vi "ParseSlaveRWw.vi"(0 "Node RWw":u16[][](array[numeric])) -> (1 "当前档位":sgl, 2 "PLC采集值":T2, 3 "PLC档位序号":T1, 4 "行号":i32)   [LabVIEW 2018]
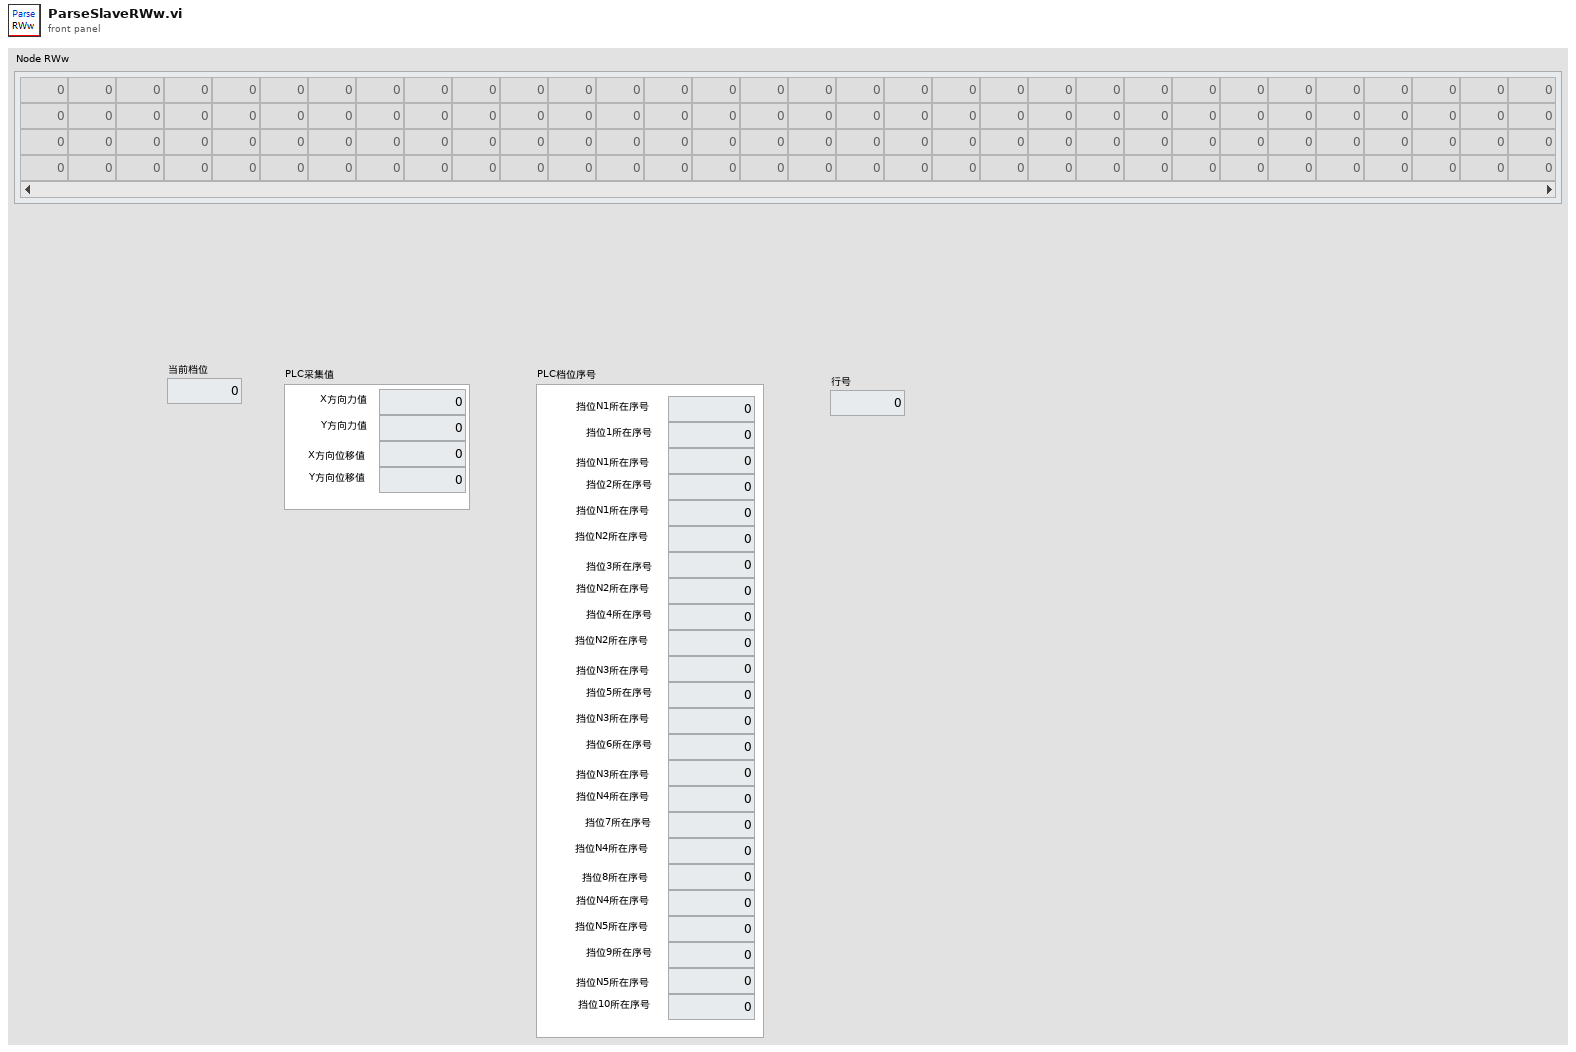
[diagram p1: front panel]
types:
  T1 = cluster{"挡位N1所在序号":sgl, "挡位1所在序号":sgl, "挡位N1所在序号":sgl, "挡位2所在序号":sgl, "挡位N1所在序号":sgl, " 挡位N2所在序号":sgl, "挡位3所在序号":sgl, "挡位N2所在序号":sgl, "挡位4所在序号":sgl, " 挡位N2所在序号":sgl, "挡位N3所在序号":sgl, "挡位5所在序号":sgl, "挡位N3所在序号":sgl, "挡位6所在序号":sgl, "挡位N3所在序号":sgl, "挡位N4所在序号":sgl, " 挡位7所在序号":sgl, " 挡位N4所在序号":sgl, "挡位8所在序号":sgl, "挡位N4所在序号":sgl, " 挡位N5所在序号":sgl, "挡位9所在序号":sgl, "挡位N5所在序号":sgl, " 挡位10所在序号":sgl}
  T2 = cluster{"X方向力值":sgl, "Y方向力值":sgl, "X方向位移值":sgl, "Y方向位移值":sgl}
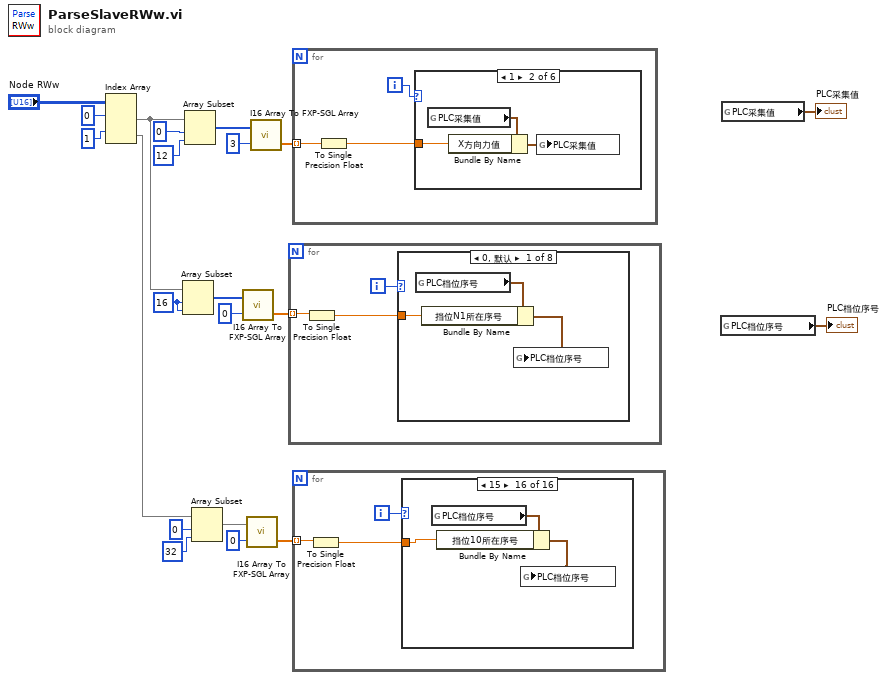
[diagram p0: block diagram]
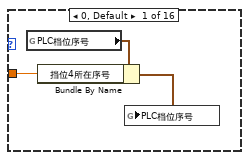
[diagram p2: hidden frame]
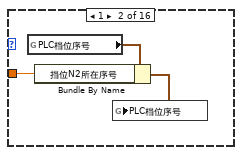
[diagram p3: hidden frame]
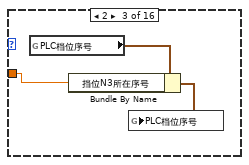
[diagram p4: hidden frame]
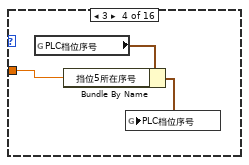
[diagram p5: hidden frame]
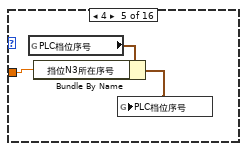
[diagram p6: hidden frame]
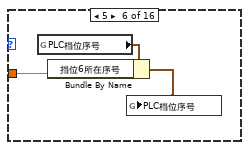
[diagram p7: hidden frame]
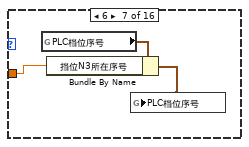
[diagram p8: hidden frame]
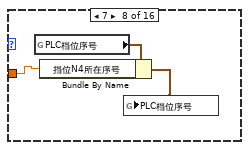
[diagram p9: hidden frame]
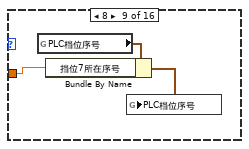
[diagram p10: hidden frame]
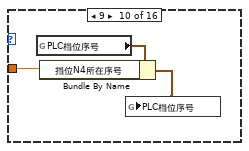
[diagram p11: hidden frame]
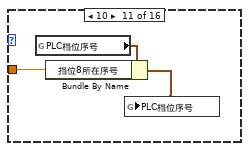
[diagram p12: hidden frame]
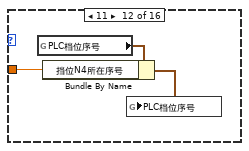
[diagram p13: hidden frame]
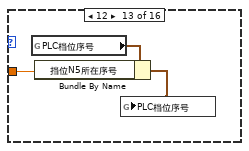
[diagram p14: hidden frame]
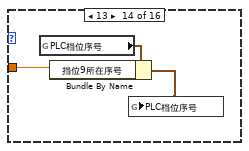
[diagram p15: hidden frame]
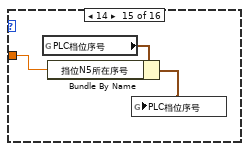
[diagram p16: hidden frame]
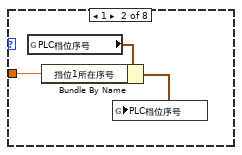
[diagram p17: hidden frame]
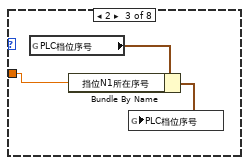
[diagram p18: hidden frame]
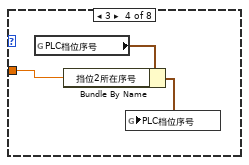
[diagram p19: hidden frame]
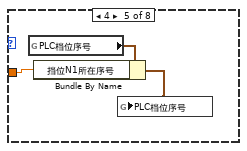
[diagram p20: hidden frame]
diagram:
  w11 = 16 ("索引")
  n1 = Index Array(array="Node RWw", index (row) #1=0 ("索引 (行)"), index (row) #2=1 ("索引 (行)")) -> (element #1=w12:u16[], element #2=w6:u16[])  [unwired: 2 in]
  n2 = Array Subset(array=w12, index=w11, length=w11) -> (w10:u16[])
  n3 = Array Subset(array=w12, index=0 ("索引"), length=12 ("长度")) -> (w15:u16[])
  n4 = Array Subset(array=w6, index=0 ("索引"), length=32 ("长度")) -> (w3:u16[])
  n5 = call "I16 Array To FXP-SGL Array.vi"("小数位数"=0, "I16 Array"=w10) -> ("SGL Array"=w8:sgl[])  [unwired: 1 out]
  n6 = call "I16 Array To FXP-SGL Array.vi"("小数位数"=0, "I16 Array"=w3) -> ("SGL Array"=w1:sgl[])  [unwired: 1 out]
  n7 = call "I16 Array To FXP-SGL Array.vi"("小数位数"=3, "I16 Array"=w15) -> ("SGL Array"=w18:sgl[])  [unwired: 1 out]
  n8 = for {
    tunnel: w8 -> [w24] mode=indexing
    i -> [w23]
    n9 = To Single Precision Float(number=w24) -> (single precision float=w22:sgl)
    n10 = case shown="0, 默认" w23 {
      tunnel: w22 -> [w26 w30 w32 w35 w39 w40 w43 w46]
      frame 0, Default {
        n11 = global read "全局 1.vi" "PLC档位序号"() -> (w27:T1)
        n12 = Bundle By Name(cluster=w27, "挡位N1所在序号"=w26) -> (w25:T1)
        n13 = global write "全局 1.vi" "PLC档位序号"(w25) -> ()
      }
      frame 1 {
        n14 = global read "全局 1.vi" "PLC档位序号"() -> (w29:T1)
        n15 = Bundle By Name(cluster=w29, "挡位1所在序号"=w30) -> (w28:T1)
        n16 = global write "全局 1.vi" "PLC档位序号"(w28) -> ()
      }
      frame 2 {
        n17 = global read "全局 1.vi" "PLC档位序号"() -> (w33:T1)
        n18 = Bundle By Name(cluster=w33, "挡位N1所在序号"=w32) -> (w31:T1)
        n19 = global write "全局 1.vi" "PLC档位序号"(w31) -> ()
      }
      frame 3 {
        n20 = global read "全局 1.vi" "PLC档位序号"() -> (w36:T1)
        n21 = Bundle By Name(cluster=w36, "挡位2所在序号"=w35) -> (w34:T1)
        n22 = global write "全局 1.vi" "PLC档位序号"(w34) -> ()
      }
      frame 4 {
        n23 = global read "全局 1.vi" "PLC档位序号"() -> (w38:T1)
        n24 = Bundle By Name(cluster=w38, "挡位N1所在序号"=w39) -> (w37:T1)
        n25 = global write "全局 1.vi" "PLC档位序号"(w37) -> ()
      }
      frame 5 {
        n26 = global read "全局 1.vi" "PLC档位序号"() -> (w42:T1)
        n27 = Bundle By Name(cluster=w42, "挡位N2所在序号"=w40) -> (w41:T1)
        n28 = global write "全局 1.vi" "PLC档位序号"(w41) -> ()
      }
      frame 6 {
        n29 = global read "全局 1.vi" "PLC档位序号"() -> (w45:T1)
        n30 = Bundle By Name(cluster=w45, "挡位3所在序号"=w43) -> (w44:T1)
        n31 = global write "全局 1.vi" "PLC档位序号"(w44) -> ()
      }
      frame 7 {
        n32 = global read "全局 1.vi" "PLC档位序号"() -> (w48:T1)
        n33 = Bundle By Name(cluster=w48, "挡位N2所在序号"=w46) -> (w47:T1)
        n34 = global write "全局 1.vi" "PLC档位序号"(w47) -> ()
      }
    }
  }
  n35 = for {
    tunnel: w18 -> [w51] mode=indexing
    i -> [w49]
    n36 = To Single Precision Float(number=w51) -> (single precision float=w50:sgl)
    n37 = case shown="1" w49 {
      tunnel: w50 -> [w54 w57 w60 w63 w66 w69]
      frame 0, Default {
        n38 = Multiply(x=w54, y=sgl 1000.0) -> (x*y=→"当前档位":sgl)
      }
      frame 1 {
        n39 = global read "全局 1.vi" "PLC采集值"() -> (w55:T2)
        n40 = Bundle By Name(cluster=w55, "X方向力值"=w57) -> (w56:T2)
        n41 = global write "全局 1.vi" "PLC采集值"(w56) -> ()
      }
      frame 2 {
        n42 = global read "全局 1.vi" "PLC采集值"() -> (w58:T2)
        n43 = Bundle By Name(cluster=w58, "Y方向力值"=w60) -> (w59:T2)
        n44 = global write "全局 1.vi" "PLC采集值"(w59) -> ()
      }
      frame 3 {
        n45 = global read "全局 1.vi" "PLC采集值"() -> (w61:T2)
        n46 = Bundle By Name(cluster=w61, "X方向位移值"=w63) -> (w62:T2)
        n47 = global write "全局 1.vi" "PLC采集值"(w62) -> ()
      }
      frame 4 {
        n48 = global read "全局 1.vi" "PLC采集值"() -> (w64:T2)
        n49 = Bundle By Name(cluster=w64, "Y方向位移值"=w66) -> (w65:T2)
        n50 = global write "全局 1.vi" "PLC采集值"(w65) -> ()
      }
      frame 5 {
        n51 = Multiply(x=w69, y=sgl 1000.0) -> (x*y=→"行号":sgl)
      }
    }
  }
  n52 = for {
    tunnel: w1 -> [w72] mode=indexing
    i -> [w71]
    n53 = To Single Precision Float(number=w72) -> (single precision float=w70:sgl)
    n54 = case shown="15" w71 {
      tunnel: w70 -> [w74 w78 w80 w83 w87 w88 w91 w94 w97 w100 w103 w106 w109 w112 w115 w118]
      frame 0, Default {
        n55 = global read "全局 1.vi" "PLC档位序号"() -> (w75:T1)
        n56 = Bundle By Name(cluster=w75, "挡位4所在序号"=w74) -> (w73:T1)
        n57 = global write "全局 1.vi" "PLC档位序号"(w73) -> ()
      }
      frame 1 {
        n58 = global read "全局 1.vi" "PLC档位序号"() -> (w77:T1)
        n59 = Bundle By Name(cluster=w77, "挡位N2所在序号"=w78) -> (w76:T1)
        n60 = global write "全局 1.vi" "PLC档位序号"(w76) -> ()
      }
      frame 2 {
        n61 = global read "全局 1.vi" "PLC档位序号"() -> (w81:T1)
        n62 = Bundle By Name(cluster=w81, "挡位N3所在序号"=w80) -> (w79:T1)
        n63 = global write "全局 1.vi" "PLC档位序号"(w79) -> ()
      }
      frame 3 {
        n64 = global read "全局 1.vi" "PLC档位序号"() -> (w84:T1)
        n65 = Bundle By Name(cluster=w84, "挡位5所在序号"=w83) -> (w82:T1)
        n66 = global write "全局 1.vi" "PLC档位序号"(w82) -> ()
      }
      frame 4 {
        n67 = global read "全局 1.vi" "PLC档位序号"() -> (w86:T1)
        n68 = Bundle By Name(cluster=w86, "挡位N3所在序号"=w87) -> (w85:T1)
        n69 = global write "全局 1.vi" "PLC档位序号"(w85) -> ()
      }
      frame 5 {
        n70 = global read "全局 1.vi" "PLC档位序号"() -> (w90:T1)
        n71 = Bundle By Name(cluster=w90, "挡位6所在序号"=w88) -> (w89:T1)
        n72 = global write "全局 1.vi" "PLC档位序号"(w89) -> ()
      }
      frame 6 {
        n73 = global read "全局 1.vi" "PLC档位序号"() -> (w93:T1)
        n74 = Bundle By Name(cluster=w93, "挡位N3所在序号"=w91) -> (w92:T1)
        n75 = global write "全局 1.vi" "PLC档位序号"(w92) -> ()
      }
      frame 7 {
        n76 = global read "全局 1.vi" "PLC档位序号"() -> (w96:T1)
        n77 = Bundle By Name(cluster=w96, "挡位N4所在序号"=w94) -> (w95:T1)
        n78 = global write "全局 1.vi" "PLC档位序号"(w95) -> ()
      }
      frame 8 {
        n79 = global read "全局 1.vi" "PLC档位序号"() -> (w99:T1)
        n80 = Bundle By Name(cluster=w99, "挡位7所在序号"=w97) -> (w98:T1)
        n81 = global write "全局 1.vi" "PLC档位序号"(w98) -> ()
      }
      frame 9 {
        n82 = global read "全局 1.vi" "PLC档位序号"() -> (w102:T1)
        n83 = Bundle By Name(cluster=w102, "挡位N4所在序号"=w100) -> (w101:T1)
        n84 = global write "全局 1.vi" "PLC档位序号"(w101) -> ()
      }
      frame 10 {
        n85 = global read "全局 1.vi" "PLC档位序号"() -> (w105:T1)
        n86 = Bundle By Name(cluster=w105, "挡位8所在序号"=w103) -> (w104:T1)
        n87 = global write "全局 1.vi" "PLC档位序号"(w104) -> ()
      }
      frame 11 {
        n88 = global read "全局 1.vi" "PLC档位序号"() -> (w108:T1)
        n89 = Bundle By Name(cluster=w108, "挡位N4所在序号"=w106) -> (w107:T1)
        n90 = global write "全局 1.vi" "PLC档位序号"(w107) -> ()
      }
      frame 12 {
        n91 = global read "全局 1.vi" "PLC档位序号"() -> (w111:T1)
        n92 = Bundle By Name(cluster=w111, "挡位N5所在序号"=w109) -> (w110:T1)
        n93 = global write "全局 1.vi" "PLC档位序号"(w110) -> ()
      }
      frame 13 {
        n94 = global read "全局 1.vi" "PLC档位序号"() -> (w114:T1)
        n95 = Bundle By Name(cluster=w114, "挡位9所在序号"=w112) -> (w113:T1)
        n96 = global write "全局 1.vi" "PLC档位序号"(w113) -> ()
      }
      frame 14 {
        n97 = global read "全局 1.vi" "PLC档位序号"() -> (w117:T1)
        n98 = Bundle By Name(cluster=w117, "挡位N5所在序号"=w115) -> (w116:T1)
        n99 = global write "全局 1.vi" "PLC档位序号"(w116) -> ()
      }
      frame 15 {
        n100 = global read "全局 1.vi" "PLC档位序号"() -> (w120:T1)
        n101 = Bundle By Name(cluster=w120, "挡位10所在序号"=w118) -> (w119:T1)
        n102 = global write "全局 1.vi" "PLC档位序号"(w119) -> ()
      }
    }
  }
  n103 = global read "全局 1.vi" "PLC档位序号"() -> (→"PLC档位序号":T1)
  n104 = global read "全局 1.vi" "PLC采集值"() -> (→"PLC采集值":T2)
